vi "Send.vi"(7 "Message Priority (Normal)":T1=enum."Normal", 8 "error in (no error)":errorcluster, 9 "Message":refnum<class "Message.lvclass">, 10 "Actor in":refnum<class "Actor.lvclass">, 11 "Sender Msg in":refnum<class "Sender Msg.lvclass">) -> (0 "error out":errorcluster, 1 "Dropped?":bool, 2 "Actor out":refnum<class "Actor.lvclass">)   [LabVIEW 2020, in "Publisher.lvlib" / "Sender Msg.lvclass"]
doc: "Send a Message somewhere through the Publisher. \nThe default implementation has no targetting so instead of sending the Sender Msg the Message is sent in a Publish Msg."
uses:
  Sender Msg.lvclass
  PPL/HDH.Actor Framework.Core.Actor.lvlibp/1abvi3w/vi.lib/ActorFramework/Message Enqueuer/Message Priority.ctl
  PPL/HDH.Actor Framework.Core.Actor.lvlibp/1abvi3w/vi.lib/ActorFramework/Message/Message.lvclass
  PPL/HDH.Actor Framework.Core.Actor.lvlibp/1abvi3w/vi.lib/ActorFramework/Actor/Actor.lvclass
  Publish Msg/Publish Msg.lvclass/Publish Msg.ctl
  Publish Msg/Publish Msg.lvclass
  C:/Current projects/WS/Framework/Framework/Actors/Publisher/Publisher Messages/Publisher Msg/Publisher Msg.lvclass
  Publisher Msg/Send To Caller.vi
  PPL/HDH.Actor Framework.Core.Actor.lvlibp/1abvi3w/vi.lib/ActorFramework/Message Enqueuer/Message Enqueuer.lvclass
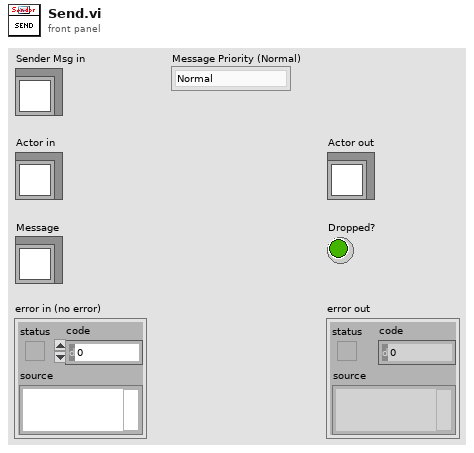
[diagram p1: front panel]
types:
  T1 = typedef "HDH.Actor Framework.Core.Actor.lvlibp/Message Enqueuer.lvclass/Message Priority.ctl" = enum16{"Low", "Normal", "High"}
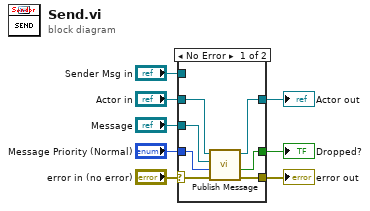
[diagram p0: block diagram]
diagram:
  n1 = case shown="No Error" "error in (no error)" {
    selector: "error in (no error)" -> [w10 w17]
    tunnel: [w9 w17] -> w7
    tunnel: "Sender Msg in" -> [_ _]
    tunnel: [w14 w16] -> w5
    tunnel: "Actor in" -> [w15 w16]
    tunnel: "Message" -> [w13 _]
    tunnel: "Message Priority (Normal)" -> [w12 _]
    tunnel: [w11 _] -> w1
    frame No Error {
      n2 = call "Publish Message.vi"("error in (no error)"=w10, "Message Priority (Normal)"=w12, "Message to Publish"=w13, "Actor in"=w15) -> ("error out"=w9:errorcluster, "Dropped?"=w11:bool, "Actor out"=w14:refnum<class "Actor.lvclass">)  [unwired: 5 in]
    }
    frame Error {
    }
  }
  "error out" <- w7
  "Actor out" <- w5
  "Dropped?" <- w1
